vi "Get UI Control Value.vi"(8 "error in (no error)":errorcluster, 10 "VI Ref":refnum<vi>, 11 "Double Parameter in":refnum<class "Double Parameter.lvclass">) -> (0 "error out":errorcluster, 3 "Double Parameter out":refnum<class "Double Parameter.lvclass">)   [LabVIEW 2016, in "CD Parameter Manager API.lvlib" / "Double Parameter.lvclass"]
uses:
  Double Parameter.lvclass
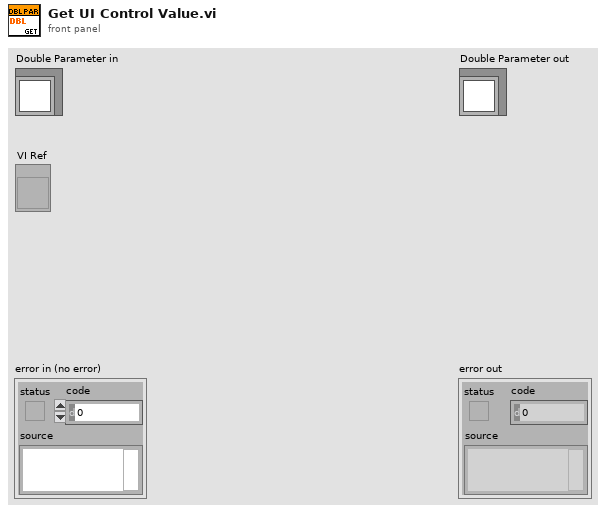
[diagram p1: front panel]
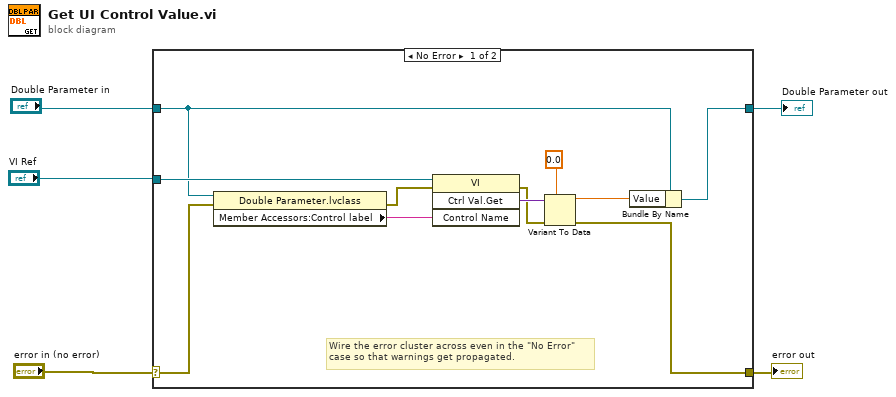
[diagram p0: block diagram]
diagram:
  n1 = case shown="No Error" "error in (no error)" {
    selector: "error in (no error)" -> [w9 w18]
    tunnel: [w6 w18] -> w5
    tunnel: [w15 w17] -> w4
    tunnel: "Double Parameter in" -> [w8 w17]
    tunnel: "VI Ref" -> [w16 _]
    frame No Error {
      # "Wire the error cluster across even in the \"No Error\"\ncase so that warnings get propagated."
      n2 = property class="Double Parameter.lvclass"(reference=w8, error in=w9) -> (error out=w10:errorcluster, "Member Accessors:Control label"=w11:string)  [unwired: 1 out]
      n3 = invoke class="VI" method="Ctrl Val.Get"(reference=w16, error in=w10, "Control Name"=w11) -> (error out=w7:errorcluster, "Get Control Value Variant"=w14:variant)  [unwired: 1 in, 2 out]
      n4 = Variant To Data(error in=w7, type=0.0 ("Value"), Variant=w14) -> (data=w13:dbl, error out=w6:errorcluster)
      n5 = Bundle By Name(cluster=w8, "Value"=w13) -> (w15:refnum<class "Double Parameter.lvclass">)
    }
    frame Error {
    }
  }
  "error out" <- w5
  "Double Parameter out" <- w4
